vi "MuxReset.vi"(8 "error in (no error)":errorcluster, 11 "KE3700A in":refnum<class "KE3706A.lvclass">) -> (0 "error out":errorcluster, 3 "KE3700A out":refnum<class "KE3706A.lvclass">)   [LabVIEW 2013, in "KE3706A.lvclass"]
uses:
  KE3706A.lvclass
  <instrlib>/Keithley 3706/Keithley 3700 Series.lvlib
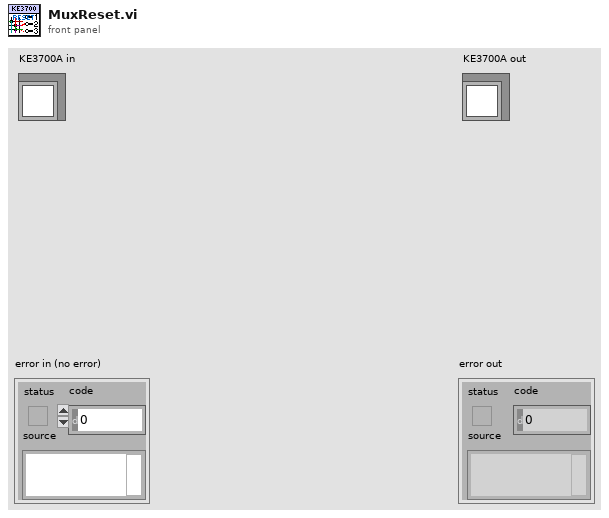
[diagram p1: front panel]
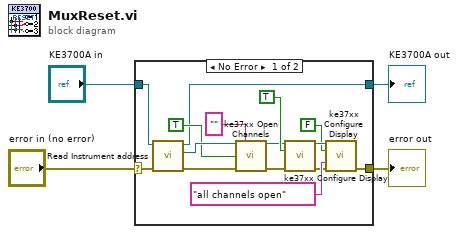
[diagram p0: block diagram]
diagram:
  n1 = case shown="No Error" "error in (no error)" {
    selector: "error in (no error)" -> [w18 w20]
    tunnel: "KE3700A in" -> [w19 w21]
    tunnel: [w13 w21] -> w2
    tunnel: [w6 w20] -> w1
    frame No Error {
      n2 = call-dynamic "Read Instrument address.vi"("error in (no error)"=w18, "InstControl in"=w19) -> ("error out"=w14:errorcluster, "VISA address"=w17:refnum<visa-resource-name>, "InstControl out"=w13:refnum<class "KE3706A.lvclass">)  [unwired: 7 in]
      n3 = call <instrlib>:"ke37xx Open Channels.vi"("VISA Resource Name"=w17, "Channel List"="", "Open All (False)"=TRUE, "error in (no error)"=w14) -> ("VISA Resource Name Out"=w5:refnum<visa-resource-name>, "error out"=w7:errorcluster)  [unwired: 10 in]
      n4 = call <instrlib>:"ke37xx Configure Display.vi"("VISA Resource Name"=w5, "Clear Display (False)"=TRUE, "error in (no error)"=w7) -> ("VISA Resource Name Out"=w11:refnum<visa-resource-name>, "error out"=w8:errorcluster)  [unwired: 11 in]
      n5 = call <instrlib>:"ke37xx Configure Display.vi"("VISA Resource Name"=w11, "Clear Display (False)"=FALSE, "Message (Empty)"="all channels open", "error in (no error)"=w8) -> ("error out"=w6:errorcluster)  [unwired: 10 in, 1 out]
    }
    frame Error {
    }
  }
  "error out" <- w1
  "KE3700A out" <- w2
